vi "SetSerial.vi"(0 "reference in":refnum<class "Test_Template.lvclass">, 5 "SN":string, 7 "BN":string, 9 "UUT_Index":i32, 11 "error in (no error)":errorcluster) -> (4 "reference in":refnum<class "Test_Template.lvclass">, 10 "OK":bool, 15 "error out":errorcluster)   [LabVIEW 2017]
uses:
  Test_Template.lvclass
  Components/TestView_Base.lvlibp/TestView_Base.lvclass
  Components/MES_Base.lvlibp/MES_Base.lvclass
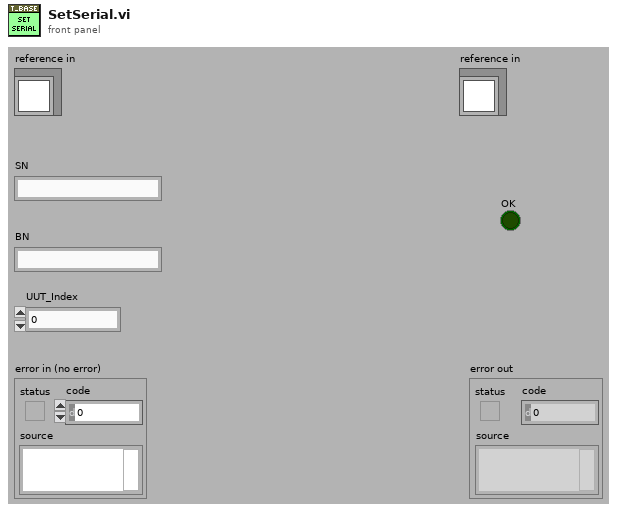
[diagram p1: front panel]
types:
  T1 = typedef "Test_Template.lvlib/Test_Template.lvclass/ObjectAttributes.ctl" = cluster{"Config":T2}
  T2 = typedef "Test_Template.lvlib/Test_Template.lvclass/Config.ctl" = cluster{"default":string}
  T3 = cluster{"Code":string, "Name":string, "Description":string, "Group":string, "IsGroup":bool, "Tag":string, "Method":string, "Parrameter":string, "DataType":enum16{"NA", "String", "Boolean", "Int", "Dbl"}, "Value":variant, "Status":enum16{"Pending", "Pass", "Fail"}, "LimitLo":variant, "LimitHi":variant, "StringMatch":string, "BooleanMatch":bool, "DisplayFormat":string, "Units":string, "TestTime":dbl}[]
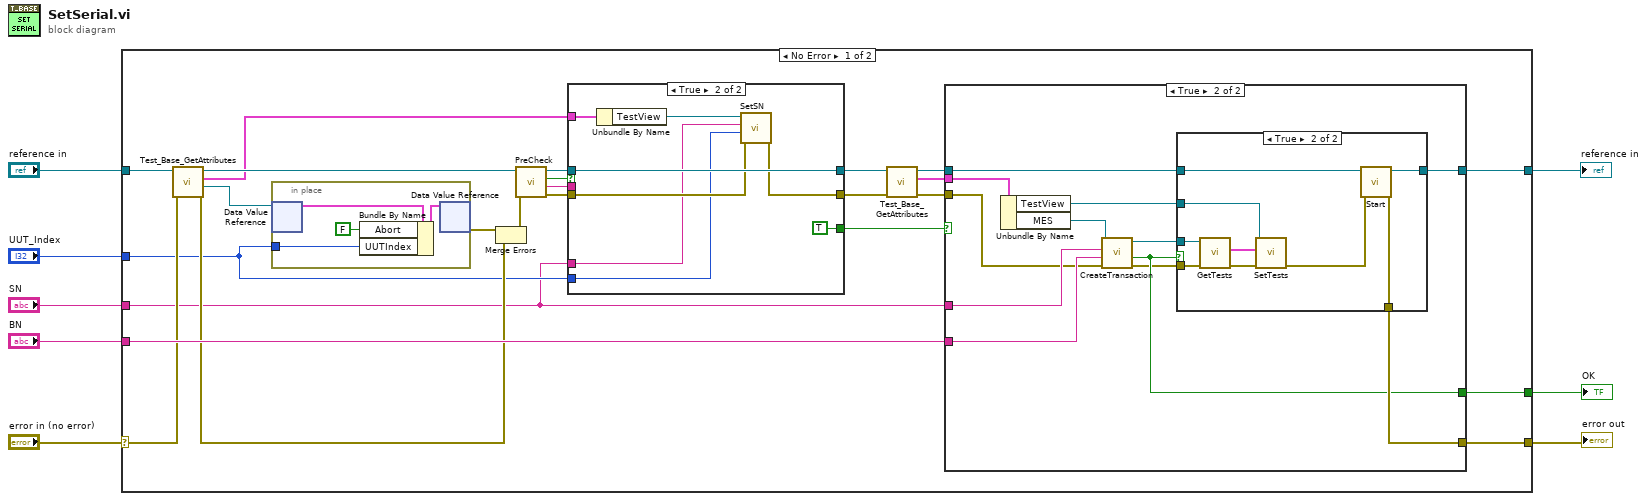
[diagram p0: block diagram]
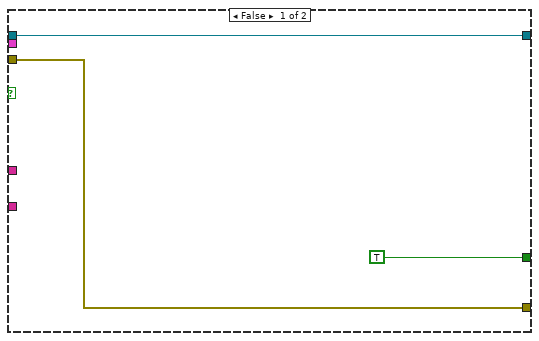
[diagram p2: hidden frame]
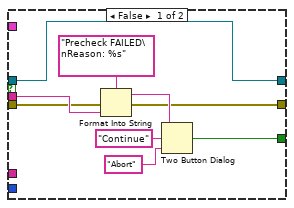
[diagram p4: hidden frame]
diagram:
  n1 = case shown="No Error" "error in (no error)" {
    selector: "error in (no error)" -> [w28 w81]
    tunnel: [w30 w81] -> w7
    tunnel: [w31 w80] -> w5
    tunnel: "reference in" -> [w29 w80]
    tunnel: "SN" -> [w9 _]
    tunnel: "BN" -> [w32 _]
    tunnel: "UUT_Index" -> [w10 _]
    tunnel: [w24 _] -> w1
    frame No Error {
      n2 = call "Test_Base_GetAttributes.vi"("error in (no error)"=w28, "reference in"=w29) -> ("error out"=w25:errorcluster, "DataRef"=w27:refnum<data-value>, "Data"=w11:T1, "reference out"=w22:refnum<class "Test_Template.lvclass">)  [unwired: 6 in]
      n3 = in-place {
        in-place-border: w10 -> [w77]
        n4 = in-place-dvr #1(w27) -> (w79:T1)  [unwired: 1 out]
        n5 = Bundle By Name(cluster=w79, "Abort"=FALSE, "UUTIndex"=w77) -> (w78:T1)
        n6 = in-place-dvr #1(w78) -> (w26:errorcluster)  [unwired: 1 out]
      }
      n7 = Merge Errors(w26, w25) -> (w23:errorcluster)
      n8 = call-dynamic "PreCheck.vi"("error in (no error)"=w23, "reference in"=w22) -> ("error out"=w21:errorcluster, "FailureMsg"=w18:string, "OK"=w20:bool, "reference in"=w19:refnum<class "Test_Template.lvclass">)  [unwired: 6 in]
      n9 = case shown="True" w20 {
        tunnel: w21 -> [w65 w71]
        tunnel: w19 -> [w59 w74]
        tunnel: w18 -> [w66 _]
        tunnel: [w61 w70] -> w15
        tunnel: [w60 TRUE ("T button?")] -> w17
        tunnel: [w59 w74] -> w13
        tunnel: w11 -> [_ w73]
        tunnel: w10 -> [_ w69]
        tunnel: w9 -> [_ w68]
        frame False {
          n10 = Format Into String(format string="Precheck FAILED\nReason: %s", error in=w65, w66) -> (resulting string=w62:string, error out=w61:errorcluster)  [unwired: 1 in]
          n11 = Two Button Dialog(message=w62, 1:"Abort" ("T button name (\"OK\")"), 2:"Continue" ("T button name (\"OK\")")) -> (T button?=w60:bool)
        }
        frame True {
          n12 = Unbundle By Name(w73) -> ("TestView"=w72:refnum<class "TestView_Base.lvclass">)
          n13 = call-dynamic "SetSN.vi"("error in (no error)"=w71, "DUT"=w69, "SN"=w68, "reference in"=w72) -> ("error out"=w70:errorcluster)  [unwired: 6 in, 1 out]
        }
      }
      n14 = call "Test_Base_GetAttributes.vi"("error in (no error)"=w15, "reference in"=w13) -> ("error out"=w16:errorcluster, "Data"=w12:T1, "reference out"=w14:refnum<class "Test_Template.lvclass">)  [unwired: 6 in, 1 out]
      n15 = case shown="True" w17 {
        tunnel: w9 -> [_ w47]
        tunnel: w32 -> [_ w46]
        tunnel: [w34 w45] -> w31
        tunnel: [w35 w44] -> w30
        tunnel: [TRUE ("OK") w43] -> w24
        tunnel: w16 -> [w35 w37]
        tunnel: w14 -> [w34 w36]
        tunnel: w12 -> [_ w38]
        frame False {
        }
        frame True {
          n16 = Unbundle By Name(w38) -> ("TestView"=w41:refnum<class "TestView_Base.lvclass">, "MES"=w40:refnum<class "MES_Base.lvclass">)
          n17 = call-dynamic "CreateTransaction.vi"("error in (no error)"=w37, "BN"=w46, "SN"=w47, "reference in"=w40) -> ("error out"=w42:errorcluster, "OK"=w43:bool, "reference in"=w39:refnum<class "MES_Base.lvclass">)  [unwired: 4 in]
          n18 = case shown="True" w43 {
            tunnel: w36 -> [w49 w56]
            tunnel: [w49 w58] -> w45
            tunnel: [w48 w57] -> w44
            tunnel: w39 -> [_ w55]
            tunnel: w42 -> [w48 w54]
            tunnel: w41 -> [_ w53]
            frame False {
            }
            frame True {
              n19 = call-dynamic "GetTests.vi"("error in (no error)"=w54, "reference in"=w55) -> ("error out"=w52:errorcluster, "Tests"=w50:T3)  [unwired: 6 in, 2 out]
              n20 = call-dynamic "SetTests.vi"("error in (no error)"=w52, "Tests"=w50, "reference in"=w53) -> ("error out"=w51:errorcluster)  [unwired: 7 in, 1 out]
              n21 = call-dynamic "Start.vi"("error in (no error)"=w51, "reference in"=w56) -> ("error out"=w57:errorcluster, "reference in"=w58:refnum<class "Test_Template.lvclass">)  [unwired: 8 in]
            }
          }
        }
      }
    }
    frame Error {
    }
  }
  "error out" <- w7
  "reference in" <- w5
  "OK" <- w1
